vi "UI (The Advanced).vi"() -> ()   [LabVIEW 2017, in "UI.lvlib"]
doc: "The Queued Message Handler of a Worker."
uses:
  UI.lvlib
  _support/Analysis Window Type.ctl
  _support/UI State.ctl
  1af51285-6659-428e-9c15-de70f1a207c9.vi
  1756710f-d813-4077-a3f9-6f06171a4225.vi
  b1498353-a107-4479-98d0-7e76c0451ff6.vi
  242d01f8-d211-4c25-bb6c-8191a2acbe42.vi
  da0d510b-1f54-4e49-9d1f-893e7e8abfcf.vi
  e403ca69-710b-4b23-8527-f02bfa86df9b.vi
  <userlib>/_NEVSTOP/Communicable State Machine(CSM)/AdvanceAPI/CSM - Revert Arguments-Safe String.vi
  <userlib>/_NEVSTOP/Communicable State Machine(CSM)/_Shared/Trim Single-line Text.vi
  <userlib>/_NEVSTOP/Communicable State Machine(CSM)/AdvanceAPI/CSM - Make String Arguments Safe.vi
  <userlib>/_NEVSTOP/Communicable State Machine(CSM)/AdvanceAPI/CSM - Break Down Multiple States String.vi
  <userlib>/_NEVSTOP/Communicable State Machine(CSM)/AdvanceAPI/CSM - Keywords.vi
  <userlib>/_NEVSTOP/Communicable State Machine(CSM)/addons/INI-Static-Variable-Support/_Support/instances/_CSM - Read File Logger Configuration - v1.0.vi
  <userlib>/_NEVSTOP/Communicable State Machine(CSM)/addons/API-String-Arugments-Support/_Support/Convert API String Arguments to Data(variant).vi
  <userlib>/_NEVSTOP/Communicable State Machine(CSM)/addons/API-String-Arugments-Support/_Support/Query Data as API String Arguments(variant).vi
  <userlib>/_NEVSTOP/Communicable State Machine(CSM)/addons/MassData-Parameter/_support/FGV-MassData(lvlibp).vi
  <userlib>/_NEVSTOP/Communicable State Machine(CSM)/_Polymophic/Add State(s) to Queue By BOOL(Element).vi
  <userlib>/_NEVSTOP/Communicable State Machine(CSM)/_Polymophic/CSM - Replace Marks in Messages.vi
  Acquisition/Acquisition.lvlib
  Logging/Logging.lvlib
  <userlib>/_NEVSTOP/Communicable State Machine(CSM)/Communicable State Machine.lvlib
  <userlib>/_NEVSTOP/Communicable State Machine(CSM)/addons/MassData-Parameter/CSM MassData Parameter Support.lvlib
  <userlib>/_NEVSTOP/Communicable State Machine(CSM)/addons/INI-Static-Variable-Support/INI-Static-Variable-Support.lvlib
  Algorithm/Algorithm.lvlib
  <userlib>/_NEVSTOP/Communicable State Machine(CSM)/addons/Logger/CSM File Logger.lvlib
  <userlib>/_NEVSTOP/Communicable State Machine(CSM)/addons/Watchdog/CSM Watchdog.lvlib
  SoundInput-DAQ/SoundInput-DAQ.lvlib
  <userlib>/_NEVSTOP/Communicable State Machine(CSM)/_Polymophic/Build Synchronous Message with Arguments.vi
panel:
  in  "Data Source":enum16{"Simulated Waveform", "Sound Card"}(ring) caption="Data Source: \nSelect Before Running"
  out "WaveformGraph":waveform(dbl)[](graph)
  in  "Analysis Window 1":T1
  out "AnalysisWnd 1":cluster{"f0":dbl, "df":dbl, "magnitude":dbl[]}[](graph)
  in  "Analysis Window 2":T1
  out "AnalysisWnd 2":cluster{"f0":dbl, "df":dbl, "magnitude":dbl[]}[](graph)
  in  "Settings":bool
  in  "Start":bool
  in  "Stop":bool
  out "Status":string
  in  "Exit":bool
  # "Continuous Measurement and Data Logger - CSM Version"
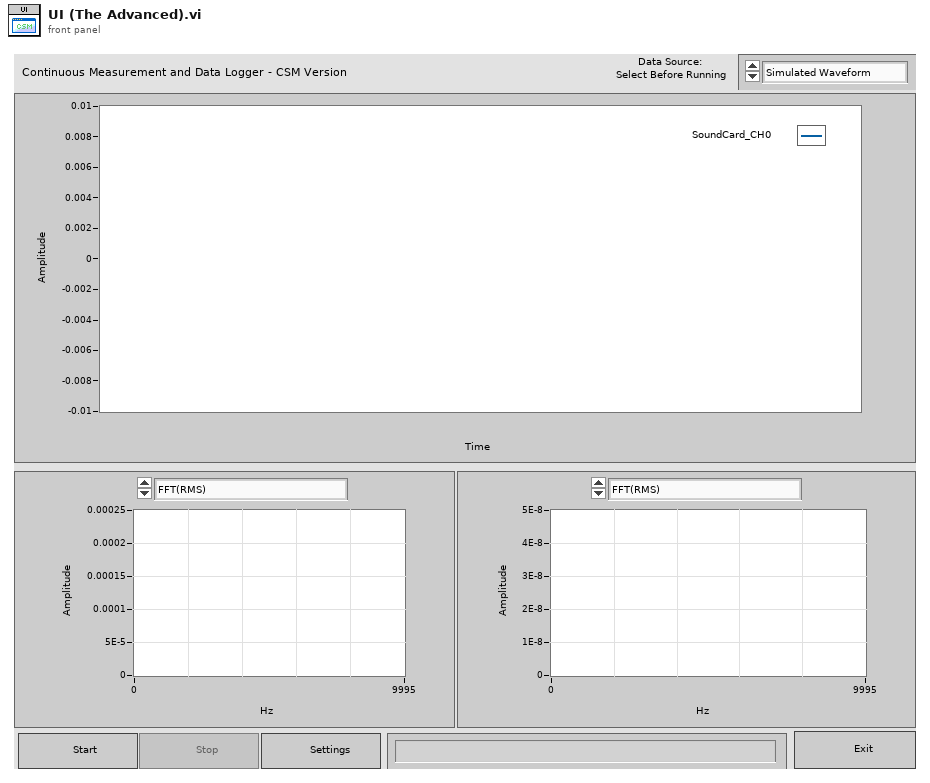
[diagram p1: front panel]
types:
  T1 = typedef "UI.lvlib/Analysis Window Type.ctl" = enum16{"FFT(RMS)", "FFT(Peak)", "Power Spectrum"}
  T2 = cluster{"Enable":bool, "Limit":cluster{"FileSize":i64, "FileNum":i32}, "Timestamp.Format":string, "AutoExit":bool}
  T3 = enum32{"Invalid", "Standard", "Closed", "Hidden", "Minimized", "Maximized"}
  T4 = enum32{"invalid app kind", "Development System", "Run Time System", "Student Edition", "Embedded LabVIEW", "Evaluation", "Custom"}
  T5 = typedef "UI.lvlib/UI State.ctl" = enum16{"Idle", "Acquiring and Logging", "Waiting for Exit", "Waiting for Exit (Acq Stopped)", "Waiting for Exit (Log Stopped)", "Waiting for Stop", "Waiting for Stop (Acq Stopped)", "Waiting for Stop (Log Stopped)"}
  T6 = enum32{"Invalid", "Default", "Floating", "Floating/Auto-Hide", "Modal"}
  T7 = typedef "Communicable State Machine.lvlib/_CSM_Response Source Message.ctl" = cluster{"‘State":string, "’Arguments":string, "’Error":errorcluster}
  T8 = cluster{"Current VI Reference":refnum<vi>, "Close Panel on Exit?":bool}
  T9 = cluster{"Core":cluster{"Current VI Reference":refnum<vi>, "Close Panel on Exit?":bool}, "UI Refs":cluster{"Start Ref":refnum<vi>, "Stop Ref":refnum<vi>, "Settings Ref":refnum<vi>, "Exit Ref":refnum<vi>, "Status Ref":refnum<vi>, "Data Ref":refnum<vi>, "Data Source Ref":refnum<vi>}, "State":T5, "Relationships":string}
  T10 = cluster{"Start Ref":refnum<vi>, "Stop Ref":refnum<vi>, "Settings Ref":refnum<vi>, "Exit Ref":refnum<vi>, "Status Ref":refnum<vi>, "Data Ref":refnum<vi>, "Data Source Ref":refnum<vi>}
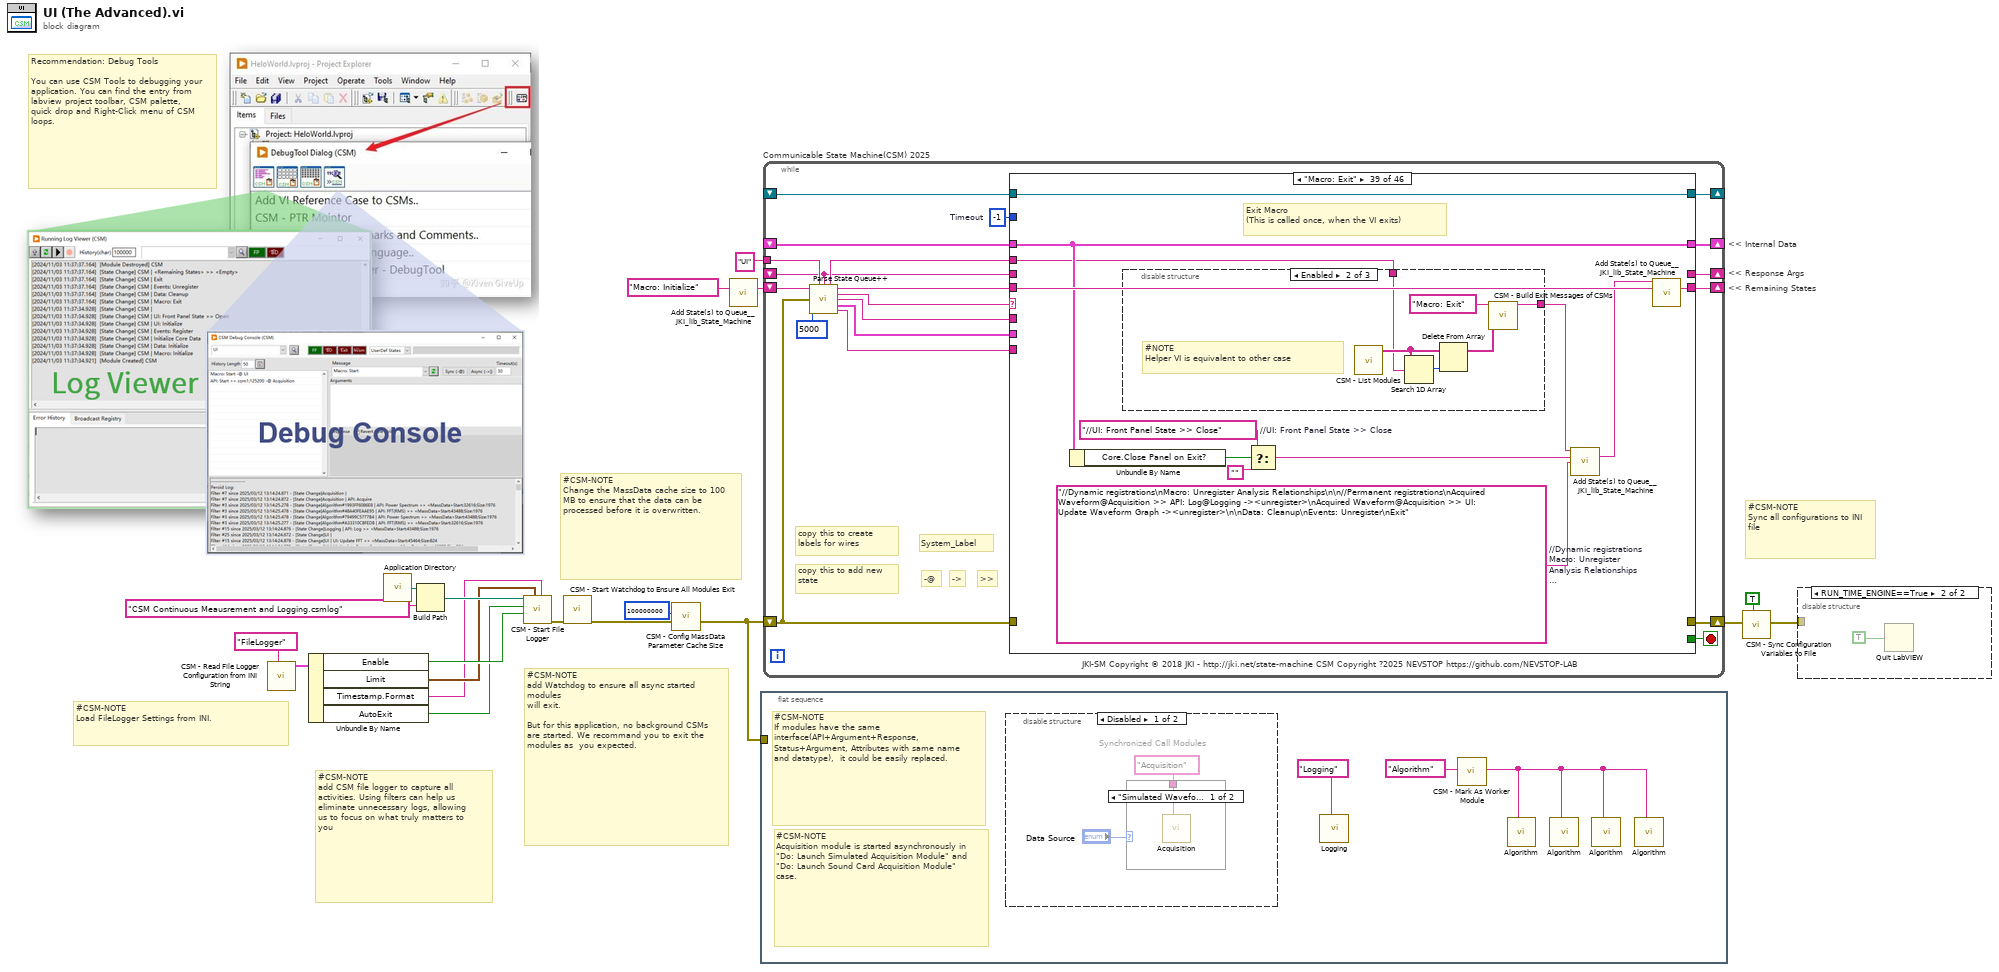
[diagram p0: block diagram]
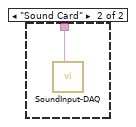
[diagram p3: hidden frame]
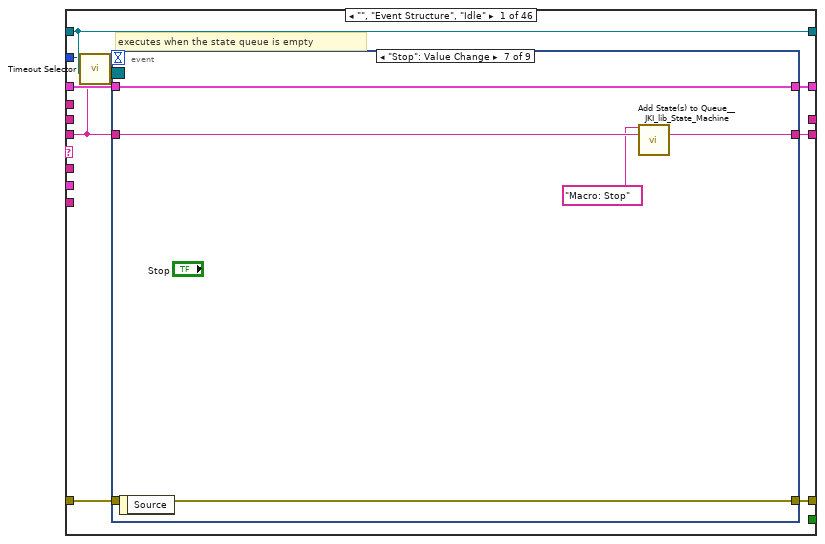
[diagram p5: hidden frame]
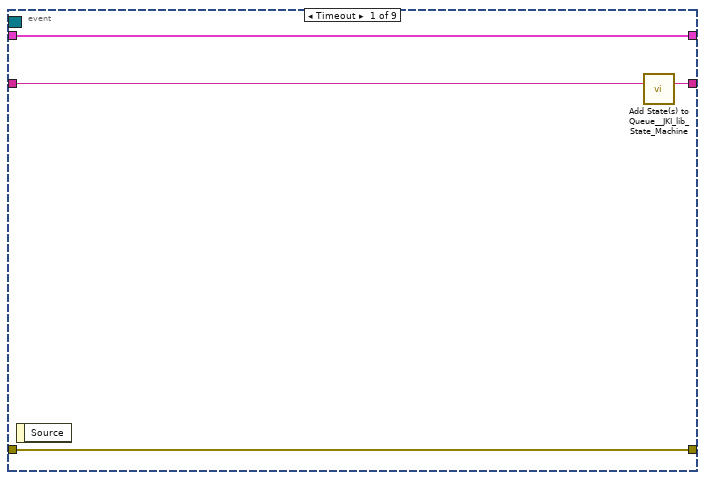
[diagram p6: hidden frame]
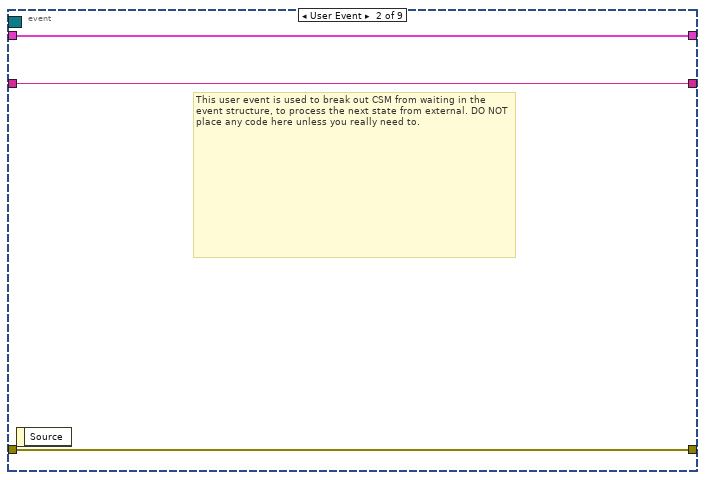
[diagram p7: hidden frame]
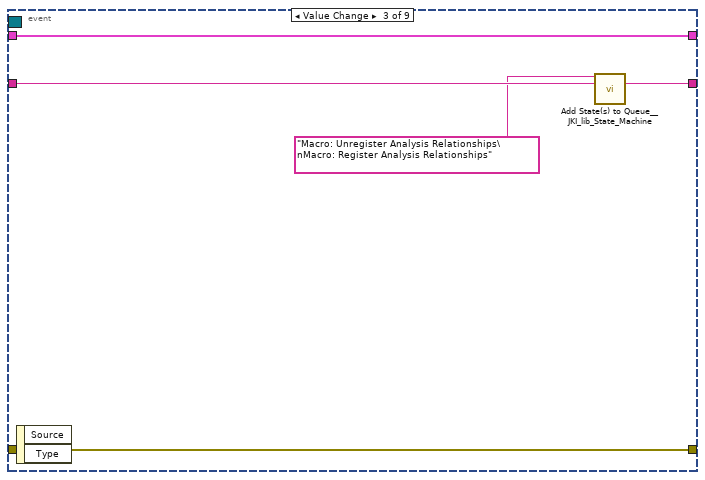
[diagram p8: hidden frame]
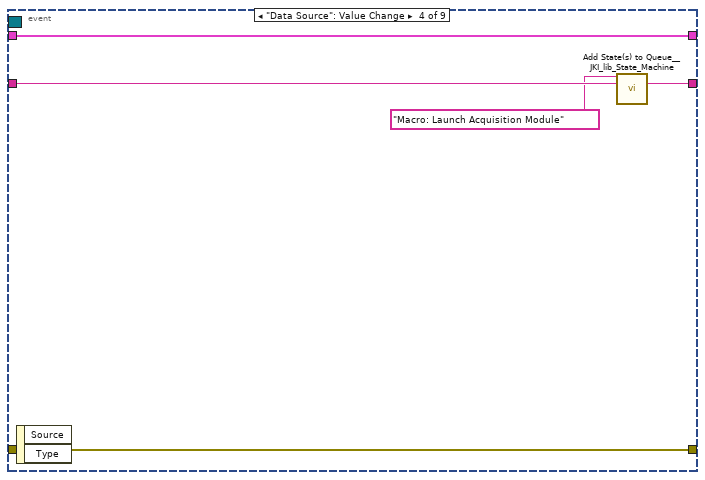
[diagram p9: hidden frame]
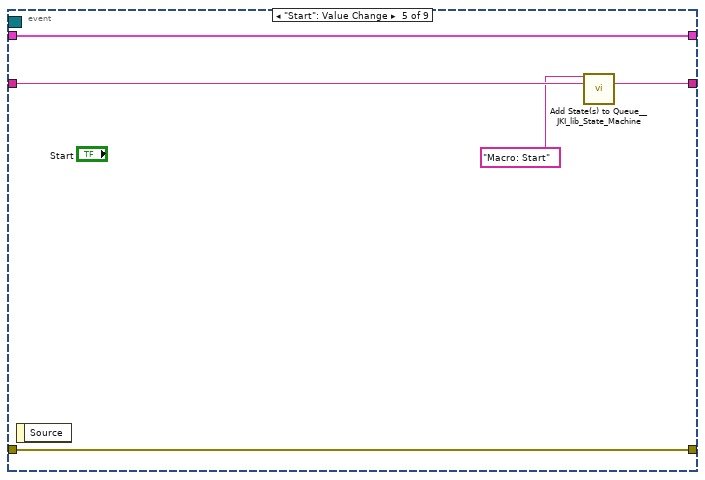
[diagram p10: hidden frame]
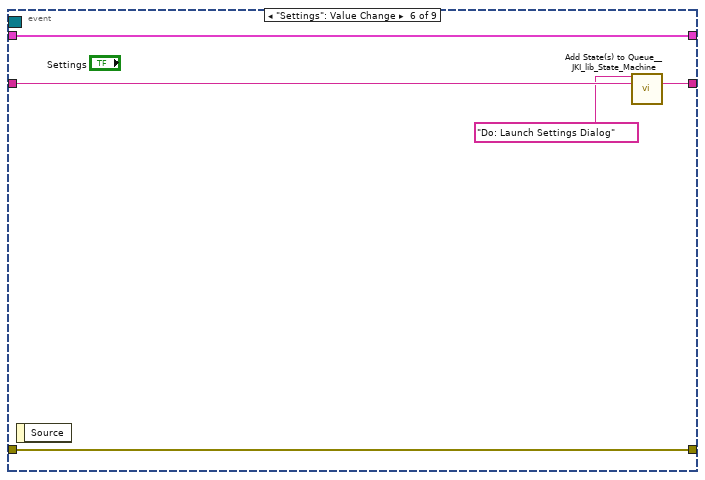
[diagram p11: hidden frame]
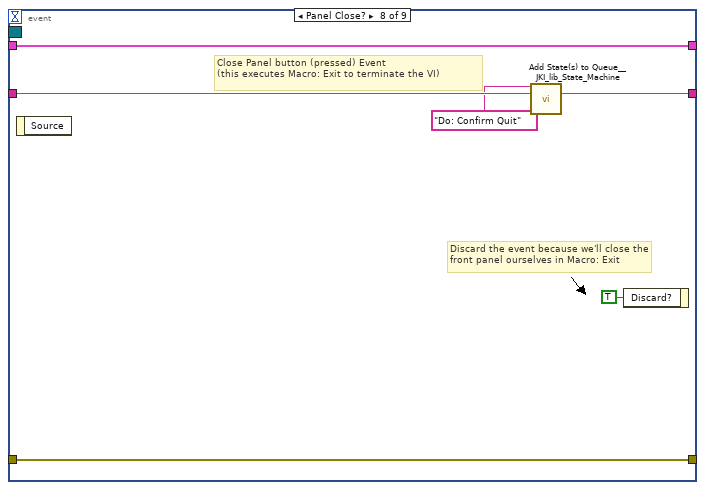
[diagram p12: hidden frame]
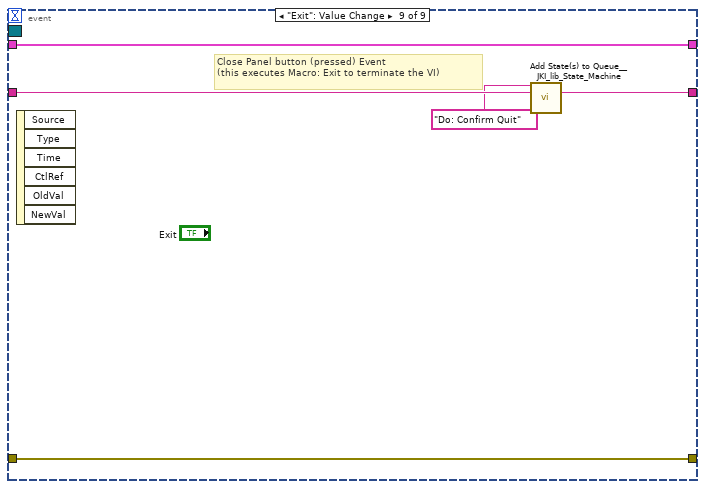
[diagram p13: hidden frame]
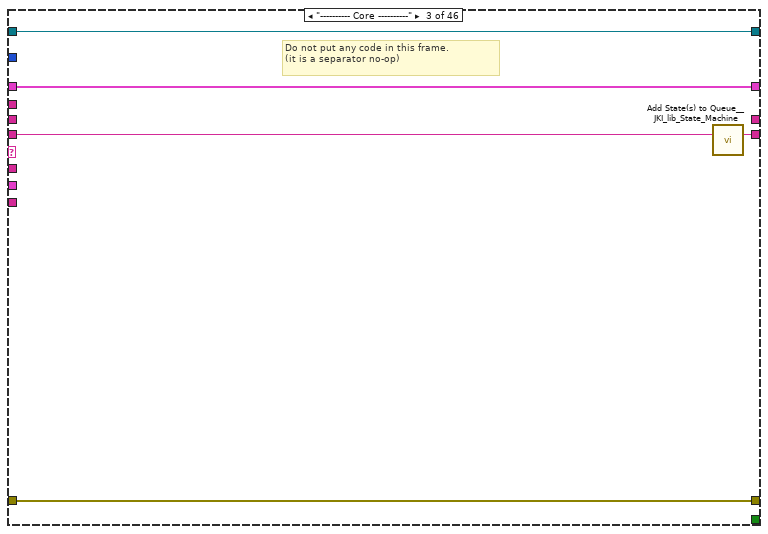
[diagram p15: hidden frame]
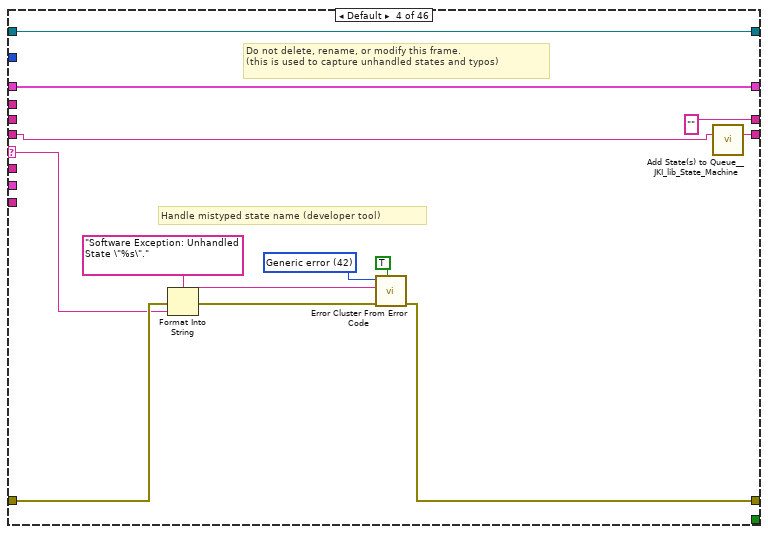
[diagram p16: hidden frame]
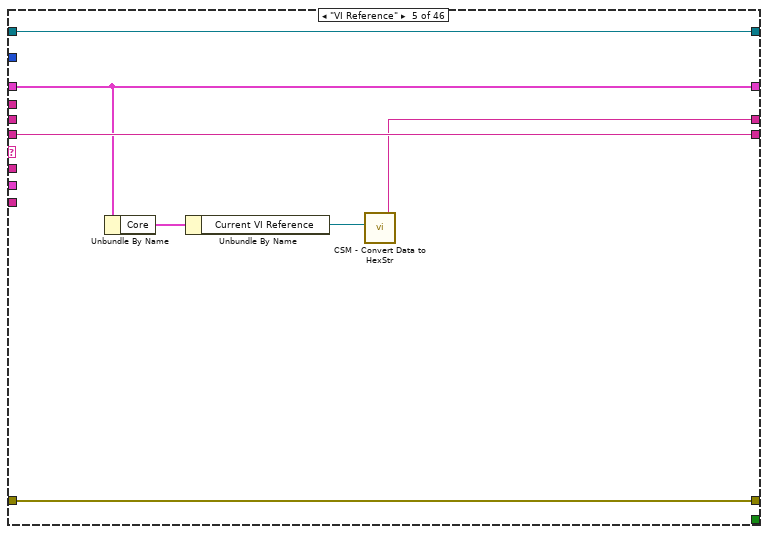
[diagram p17: hidden frame]
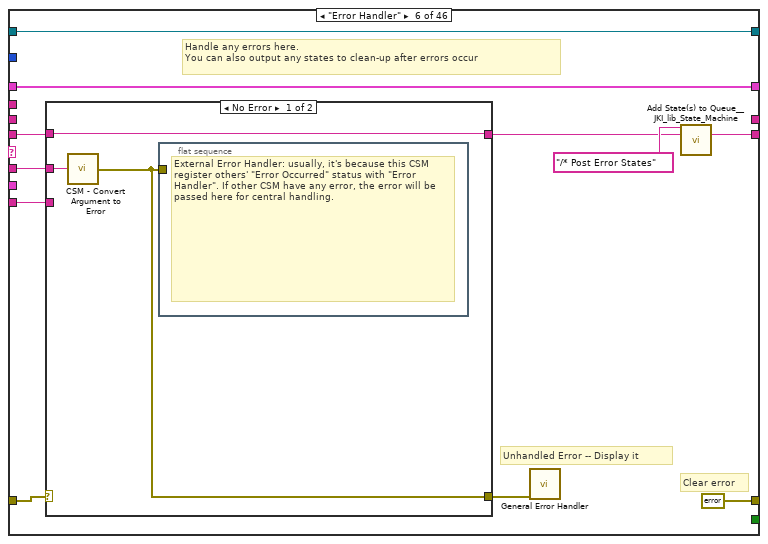
[diagram p18: hidden frame]
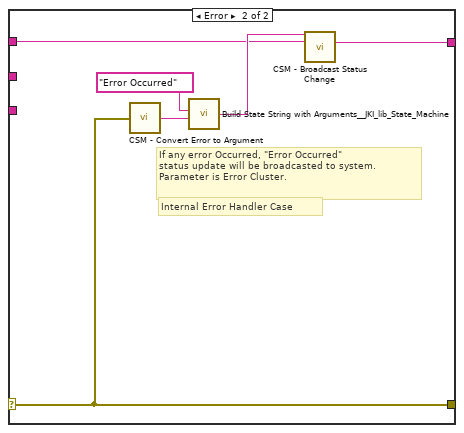
[diagram p19: hidden frame]
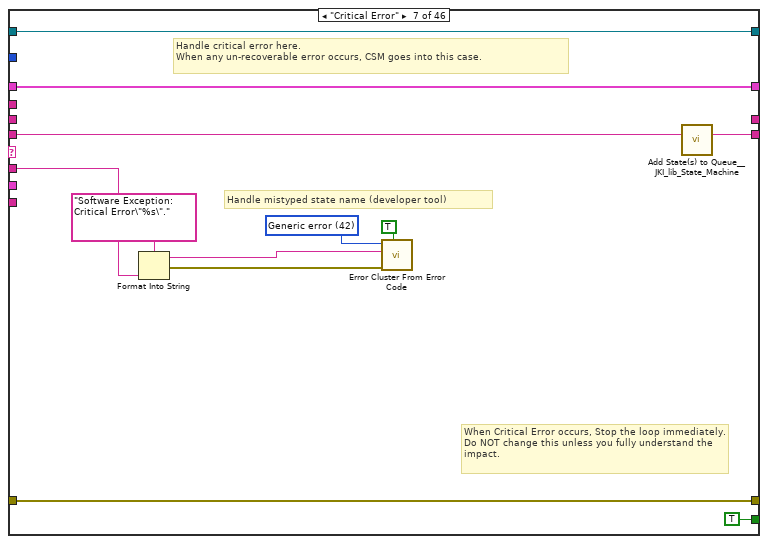
[diagram p20: hidden frame]
diagram:
  # "#CSM-NOTE\nSync all configurations to INI file"
  # "#CSM-NOTE\nChange the MassData cache size to 100 MB to ensure that the data can be processed before it is overwritten."
  # "Recommendation: Debug Tools\n\nYou can use CSM Tools to debugging your application. You can find the entry from labview project toolbar, CSM palette, quick drop and Right-Click menu of CSM loops."
  # "#CSM-NOTE\nLoad FileLogger Settings from INI."
  # "#CSM-NOTE\nadd CSM file logger to capture all activities. Using filters can help us eliminate unnecessary logs, allowing us to focus on what truly matters to you"
  # "#CSM-NOTE\nadd Watchdog to ensure all async started modules\nwill exit. \n\nBut for this application, no background CSMs are started. We recommand you to exit the modules as  you expected."
  # "<< Internal Data"
  # "<< Response Args"
  # "<< Remaining States"
  n1 = call-poly <userlib>:"CSM - Read File Logger Configuration from INI String.vi"("Section Name(\"FileLogger\")"="FileLogger" ("Section Name(\"\" as Default)")) -> ("FileLogger Configuration-v1"=w11:T2)  [unwired: 7 in, 1 out]
  n2 = Unbundle By Name(w11) -> ("Enable"=w10:bool, "Limit"=w9:cluster{"FileSize":i64, "FileNum":i32}, "Timestamp.Format"=w7:string, "AutoExit"=w8:bool)
  n3 = call <vilib>:"Application Directory.vi"() -> ("Application Directory"=w16:path)
  n4 = Build Path(base path=w16, name or relative path="CSM Continuous Meausrement and Logging.csmlog") -> (appended path=w14:path)
  n5 = call <userlib>:"CSM - Start File Logger.vi"("Timestamp Format"=w7, "Log Limit"=w9, "Watchdog? (T)"=w10, "Exit When All Module Exist? (F)"=w8, "Log File Path"=w14) -> ("error out"=w13:errorcluster)  [unwired: 4 in, 2 out]
  n6 = call <userlib>:"CSM - Start Watchdog to Ensure All Modules Exit.vi"("error in (no error)"=w13) -> ("error out"=w5:errorcluster)  [unwired: 10 in]
  n7 = call <userlib>:"CSM - Config MassData Parameter Cache Size.vi"("Error in"=w5, "Size (50M)"=100000000 ("size(1M)")) -> ("Error out"=w4:errorcluster)  [unwired: 9 in]
  n8 = call <vilib>:"Add State(s) to Queue__JKI_lib_State_Machine.vi"("State(s) in (\"\")"="Macro: Initialize") -> ("States Out"=w17:string)  [unwired: 14 in]
  n9 = flat-sequence {
    tunnel: w4 -> [_]
    frame #0 {
      # "#CSM-NOTE\nAcquisition module is started asynchronously in \"Do: Launch Simulated Acquisition Module\" and \"Do: Launch Sound Card Acquisition Module\" case."
      # "#CSM-NOTE\nIf modules have the same interface(API+Argument+Response, Status+Argument, Attributes with same name and datatype),  it could be easily replaced."
      n10 = disable-structure shown="Disabled" {
        frame Disabled {
          # "Synchronized Call Modules"
          n11 = case shown="\"Simulated Waveform\", Default" "Data Source" {
            tunnel: "Acquisition" ("Name(\"\" to use uuid)") -> [w25 w26]
            frame "Simulated Waveform", Default {
              n12 = call "Acquisition.vi"("Name(\"\" to use uuid)"=w25) -> ()  [unwired: 11 in]
            }
            frame "Sound Card" {
              n13 = call "SoundInput-DAQ.vi"("Name(\"\" to use uuid)"=w26) -> ()  [unwired: 11 in]
            }
          }
        }
        frame Enabled {
        }
      }
      n14 = call "Logging.vi"("Name(\"\" to use uuid)"="Logging" ("Name(\"\" to use uuid)")) -> ()  [unwired: 11 in]
      n15 = call <userlib>:"CSM - Mark As Worker Module.vi"("CSM Name"="Algorithm" ("Name(\"\" to use uuid)")) -> ("CSM Name (Marked As Worker)"=w20:string)  [unwired: 9 in]
      n16 = call "Algorithm.vi"("Name(\"\" to use uuid)"=w20) -> ()  [unwired: 11 in]
      n17 = call "Algorithm.vi"("Name(\"\" to use uuid)"=w20) -> ()  [unwired: 11 in]
      n18 = call "Algorithm.vi"("Name(\"\" to use uuid)"=w20) -> ()  [unwired: 11 in]
      n19 = call "Algorithm.vi"("Name(\"\" to use uuid)"=w20) -> ()  [unwired: 11 in]
    }
  }
  n20 = while "Communicable State Machine(CSM) 2025" {
    shift-right: [w41] -> _
    shift-left: _ -> [w40]
    shift-right: [w44] -> w2
    shift-left: w4 -> [w38]
    shift-right: [w43] -> _
    shift-left: w17 -> [w45]
    tunnel: "UI" ("Name(\"\" to use uuid)") -> [w33]
    shift-right: [w36] -> _
    shift-left: _ -> [w28]
    shift-right: [w35] -> _
    shift-left: _ -> [w34]
    stop <- w42 stop-if-true
    w39 = -1  # Timeout
    # "JKI-SM Copyright © 2018 JKI - http://jki.net/state-machine CSM Copyright ?2025 NEVSTOP https://github.com/NEVSTOP-LAB"
    # "copy this to add new state"
    # ">>"
    # "->"
    # "-@"
    # "copy this to create labels for wires"
    # "System_Label"
    n21 = call <userlib>:"Parse State Queue++.vi"("State Queue"=w45, "Name (\"\" to Use UUID)"=w33, "Response Arguments"=w28, "Previous Error"=w38, "Response Timeout (-2 Use Global Settings)"=5000 ("Response Timeout(1000ms)")) -> ("Name Used"=w29:string, "Remaining States"=w46:string, "Current State"=w32:string, "Arguments"=w27:string, "Additional Information"=w31:T7, "Source CSM"=w30:string)  [unwired: 5 in]
    n22 = case shown="\"Macro: Exit\"" w32 {
      selector: w32 -> [_ _ _ w110 _ _ _ _ _ _ _ _ _ _ _ _ _ _ _ _ _ _ _ _ _ _ _ _ _ _ _ _ _ _ _ _ _ _ _ _ _ _ _ _ _ _]
      tunnel: w46 -> [w47 w101 w107 w114 w126 w131 w157 w167 w180 w188 w192 w207 w214 w219 w228 w234 w241 w248 w253 w259 w263 w269 w290 w302 w315 w323 w339 w413 w422 w435 w442 w447 w454 w459 w473 w481 w492 w503 w521 w546 w552 w560 w598 w623 w644 w659]
      tunnel: w27 -> [_ _ _ _ _ w129 w150 w163 w176 _ _ _ _ _ _ w232 w238 _ _ _ _ _ _ _ _ w318 w333 w408 w426 w432 w439 _ _ _ _ _ _ _ _ _ w547 _ _ _ _ _]
      tunnel: w40 -> [w54 w100 w104 w112 w125 w137 w158 w165 w178 w187 w191 w200 w212 w216 _ w231 w239 w243 w250 w258 w262 w266 w276 w292 w305 w321 w335 w411 w428 w434 w441 w444 w451 w462 w476 w488 w495 w499 w519 w543 w549 w553 w593 w622 w643 w658]
      tunnel: [w53 w102 w105 w116 w127 errorcluster {"status"=FALSE, "code"=0, "source"=""} ("error out") w159 errorcluster {"status"=FALSE, "code"=0, "source"=""} ("error out") errorcluster {"status"=FALSE, "code"=0, "source"=""} ("error out") w189 w193 w204 w211 w217 w222 w230 w237 w244 w251 w254 w261 w267 w288 w303 w316 w319 w336 w405 w424 w431 w438 w445 w452 w463 w477 w490 w498 w507 _ w544 w550 w554 _ w615 w631 w646] -> w44
      tunnel: w38 -> [w52 w102 w105 w115 w127 w135 w159 w168 w181 w189 w193 w204 w211 w217 w222 _ _ w245 w251 _ w264 w267 w288 w303 w316 w320 w337 _ _ _ _ w445 w452 w463 w477 w490 w498 w507 _ w544 w550 _ _ _ _ _]
      tunnel: [w55 w101 w106 w113 w126 w133 w156 w166 w179 w188 w192 w206 w213 w218 w227 w234 w241 w247 w252 w259 w263 w268 w289 w302 w315 w322 w338 w413 w423 w435 w442 w446 w453 w460 w474 w482 w493 w504 w520 w545 w551 w560 w591 w623 w644 w659] -> w43
      tunnel: [_ _ _ _ _ _ TRUE _ _ _ _ _ TRUE _ _ _ _ _ _ _ _ _ _ _ _ _ _ _ _ _ _ _ _ _ _ _ _ _ _ _ _ _ _ _ _ _] -> w42
      tunnel: [w51 w100 w104 w112 w125 w137 w158 w165 w178 w187 w191 w205 w212 w216 w221 w229 w235 w243 w250 w258 w262 w266 w275 w292 w305 w321 w335 w411 w428 w434 w441 w444 w451 w462 w472 w479 w494 w505 w519 w543 w549 w553 w592 w622 w643 w658] -> w41
      tunnel: w39 -> [w49 _ _ _ _ _ _ _ _ _ _ _ _ _ _ _ _ _ _ _ _ _ _ _ _ _ _ _ _ _ _ _ _ _ _ _ _ _ _ _ _ _ _ _ _ _]
      tunnel: w30 -> [_ _ _ _ _ w128 _ _ _ _ _ _ _ _ _ _ _ _ _ _ _ _ _ _ _ _ _ _ _ _ _ _ _ _ _ _ _ _ _ _ _ _ _ _ _ _]
      tunnel: w31 -> [_ _ _ _ _ _ _ _ _ _ _ _ _ _ _ _ _ _ _ _ _ _ _ _ _ _ _ _ _ _ _ _ _ _ _ _ _ _ _ _ _ _ _ _ _ _]
      tunnel: [_ _ _ "" w121 _ _ _ _ _ _ _ _ _ _ _ w236 _ _ _ _ _ _ _ _ _ _ _ _ _ _ _ _ _ _ _ _ _ _ _ _ _ _ _ _ _] -> w36
      tunnel: [w50 w99 w103 w108 w124 w136 w148 w162 w175 w186 w190 w194 w209 w215 w225 w233 w240 w242 w249 w257 w260 w265 w287 w301 w314 w317 w332 w412 w427 w433 w440 w443 w450 w461 w475 w489 w497 w506 w512 w542 w548 w561 w597 w621 w642 w657] -> w35
      tunnel: w34 -> [w50 w99 w103 w108 w124 w136 w148 w162 w175 w186 w190 w194 w209 w215 w225 w233 w240 w242 w249 _ w260 w265 w287 w301 w314 w317 w332 w412 w427 w433 w440 w443 w450 w461 w475 w489 w497 w506 w512 w542 w548 w561 w597 w621 w642 w657]
      tunnel: w29 -> [_ _ _ _ _ _ _ _ _ _ _ _ _ _ _ _ _ _ _ w256 _ _ _ _ _ _ _ _ _ _ _ _ _ _ _ _ _ _ w510 _ _ w556 _ w618 _ _]
      tunnel: w28 -> [_ _ _ _ _ _ _ _ _ _ _ _ _ _ _ _ _ _ _ _ _ _ _ _ _ _ _ _ _ _ _ _ _ _ _ _ _ _ _ _ _ _ _ _ _ _]
      frame "", "Event Structure", "Idle" {
        # "executes when the state queue is empty"
        n23 = call <userlib>:"Timeout Selector.vi"("Remaining States"=w47, "Timeout Expected"=w49) -> ("Timeout"=w48:i32)  [unwired: 5 in]
        n24 = event shown="[6] \"Stop\": Value Change" {
          selector: w50 -> [_ _ _ _ _ _ _ _ _]
          dyn-events: _ -> [_ _ _ _ _ _ _ _ _]
          timeout: w48 -> [_ _ _ _ _ _ _ _ _]
          tunnel: w47 -> [w59 w61 w64 w69 w74 w79 w84 w93 w98]
          tunnel: [w58 w61 w65 w70 w75 w80 w85 w92 w97] -> w55
          tunnel: w54 -> [w56 w62 w66 w71 w76 w81 w86 w90 w95]
          tunnel: [w57 w60 w67 w72 w77 w82 w87 w91 w96] -> w53
          tunnel: w52 -> [w57 w60 w67 w72 w77 w82 w87 w91 w96]
          tunnel: [w56 w62 w66 w71 w76 w81 w86 w90 w95] -> w51
          event Timeout {
            n25 = event-data() -> ()  [unwired: 1 in, 1 out]
            n26 = call <vilib>:"Add State(s) to Queue__JKI_lib_State_Machine.vi"("State(s) in (\"\")"=w59) -> ("States Out"=w58:string)  [unwired: 14 in]
          }
          event User Event {
            # "This user event is used to break out CSM from waiting in the event structure, to process the next state from external. DO NOT place any code here unless you really need to."
            n27 = event-data() -> ()  [unwired: 1 in, 1 out]
          }
          event Value Change {
            n28 = event-data() -> ()  [unwired: 1 in, 2 out]
            n29 = call <vilib>:"Add State(s) to Queue__JKI_lib_State_Machine.vi"("State(s) in Front (\"\")"="Macro: Unregister Analysis Relationships\nMacro: Register Analysis Relationships" ("State(s) in Front (\"\")"), "State(s) in (\"\")"=w64) -> ("States Out"=w65:string)  [unwired: 13 in]
          }
          event "Data Source": Value Change {
            n30 = event-data() -> ()  [unwired: 1 in, 2 out]
            n31 = call <vilib>:"Add State(s) to Queue__JKI_lib_State_Machine.vi"("State(s) in Front (\"\")"="Macro: Launch Acquisition Module" ("State(s) in Front (\"\")"), "State(s) in (\"\")"=w69) -> ("States Out"=w70:string)  [unwired: 13 in]
          }
          event "Start": Value Change {
            n32 = event-data() -> ()  [unwired: 1 in, 1 out]
            n33 = call <vilib>:"Add State(s) to Queue__JKI_lib_State_Machine.vi"("State(s) in Front (\"\")"="Macro: Start" ("State(s) in Front (\"\")"), "State(s) in (\"\")"=w74) -> ("States Out"=w75:string)  [unwired: 13 in]
          }
          event "Settings": Value Change {
            n34 = event-data() -> ()  [unwired: 1 in, 1 out]
            n35 = call <vilib>:"Add State(s) to Queue__JKI_lib_State_Machine.vi"("State(s) in Front (\"\")"="Do: Launch Settings Dialog" ("State(s) in Front (\"\")"), "State(s) in (\"\")"=w79) -> ("States Out"=w80:string)  [unwired: 13 in]
          }
          event "Stop": Value Change {
            n36 = event-data() -> ()  [unwired: 1 in, 1 out]
            n37 = call <vilib>:"Add State(s) to Queue__JKI_lib_State_Machine.vi"("State(s) in Front (\"\")"="Macro: Stop" ("State(s) in Front (\"\")"), "State(s) in (\"\")"=w84) -> ("States Out"=w85:string)  [unwired: 13 in]
          }
          event Panel Close? {
            # "Discard the event because we'll close the front panel ourselves in Macro: Exit"
            # "Close Panel button (pressed) Event\n(this executes Macro: Exit to terminate the VI)"
            n38 = event-data() -> ()  [unwired: 1 in, 1 out]
            n39 = call <vilib>:"Add State(s) to Queue__JKI_lib_State_Machine.vi"("State(s) in Front (\"\")"="Do: Confirm Quit", "State(s) in (\"\")"=w93) -> ("States Out"=w92:string)  [unwired: 13 in]
            n40 = event-data("Discard?"=TRUE) -> ()  [unwired: 1 in, 1 out]
          }
          event "Exit": Value Change {
            # "Close Panel button (pressed) Event\n(this executes Macro: Exit to terminate the VI)"
            n41 = event-data() -> ()  [unwired: 1 in, 6 out]
            n42 = call <vilib>:"Add State(s) to Queue__JKI_lib_State_Machine.vi"("State(s) in Front (\"\")"="Do: Confirm Quit", "State(s) in (\"\")"=w98) -> ("States Out"=w97:string)  [unwired: 13 in]
          }
        }
      }
      frame "CSM Documentation" {
        # "CSM Documentation"
        # "State Syntax:\nStateCategory: State >> Argument -@ CSMName\nStateCategory: State >> Argument -> CSMName\n\nLine Terminator: Line feed"
        # "Commenting:\nTo add a comment use \"//\" or \"#\" and all text to the right will be ignored\nCommenting Example:\nUI: Initialize // This initializes the UI\n// Another comment line"
        # "Example:\nUI: Help >> About -@Main\nUI: Help >> About ->Main\n\nWhere \"UI\" is the state category\nWhere \"Help\" is the state\nWhere \"About\" is the argument\nWhere \"Main\" is the Name of CSM,which actually run the \"UI: Help >> About\"\n\n    \"-@\" stands for sync state. Current CSM will wait until the state is finished. \n            - if \"Main\" named CSM does not exist, \"Target Error\" will occur.\n            - if \"Main\" named CSM is in another sync remote state, \"Target Busy Error\" will occur.\n            - if \"Main\" named CSM could not finish the state in time, \"Target Timeout Error\" will occur.\n            - if everything is right. \"Response\" will occur with Argument back from \"Main\" named CSM. \n\n    \"->\" stands for async state. Current CSM will post the state and continue to next state in next iteration.\n            - if \"Main\" named CSM does not exist, \"Target Error\" will occur.\n            - if everything is right. \"Async Message Posted\" will occur.\n            - After State is finished. Caller will receive a \"Async Response\" state from callee.\n\nWhen duplicated name is used for multiple CSM module or some framework problem happens, \"Critical Error\" will occur."
      }
      frame "---------- Core ----------" {
        # "Do not put any code in this frame.\n(it is a separator no-op)"
        n43 = call <vilib>:"Add State(s) to Queue__JKI_lib_State_Machine.vi"("State(s) in (\"\")"=w107) -> ("States Out"=w106:string)  [unwired: 14 in]
      }
      frame Default {
        w119 = 42 items=["No error", "Argument error", "Memory is full", "Out of zone", "End of file", "File already open", "Generic file I/O error", "File not found", "File permission error", "Disk is full", "Duplicate path", "Too many files open", "System feature not enabled", "Resource file not found", "Cannot add resource", "Resource not found", "Image not found", "Image memory error", "Pen does not exist", "Config type invalid", "Config token not found", "Config parse error", "Config memory error", "Bad external code format", "Bad external code offset", "External code not present", "Null window", "Destroy window error", "Null menu", "Print aborted", "Bad print record", "Print driver error", "Windows error during printing", "Memory error during printing", "Print dialog error", "Generic print error", "Invalid device refnum", "Device not found", "Device parameter error", "Device unit error", "Cannot open device", "Device call aborted", "Generic error", "Cancelled by user", "Object ID too low", "Object ID too high", "Object not in heap", "Unknown heap", "Unknown object (invalid DefProc)", "Unknown object (DefProc not in table)", "Message out of range", "Invalid (null) method", "Unknown message", "Manager call not supported", "Bad address", "Network operation in progress", "Network operation timed out", "Connection is busy", "Network attribute not supported", "Network error", "Address in use", "System out of memory", "Connection aborted", "Connection refused", "Not connected", "Already connected", "Connection closed", "Initialization error (interapplication manager)", "Bad occurrence", "Wait on unbound occurrence handler", "Occurrence queue overflow", "Datalog type conflict", "Unused", "Unrecognized type (interapplication manager)", "Memory corrupt", "Failed to make temporary DLL", "Old CIN version", "Drag socket not found", "Failed to load drop-object", "Failed to register OLE object", "Failed to release OLE object", "Format specifier type mismatch", "Unknown format specifier", "Too few format specifiers", "Too many format specifiers", "Scan failed", "Newer CIN version", "Error converting to variant", "Runtime menu error", "Password tampered", "Variant attribute not found", "Incompatible variant data type", "Event data is not available", "Event Store is not present", "Occurrence is not found", "Event Queue is not created", "Event info is not available", "Refnum passed is NULL", "Error retrieving Class GUID", "Error retrieving CoClass GUID", "Error retrieving TypeLib GUID.", "Bad built application magic bytes.", "Specific driver is different from the specific driver associated with the Logical Name.", "There is no session opened to the class driver.", "Max Error", "MAX - Error with config objects", "MAX - Error loading configuration", "MAX - Group not supported"]
        # "Do not delete, rename, or modify this frame.\n(this is used to capture unhandled states and typos)"
        # "Handle mistyped state name (developer tool)"
        n44 = Format Into String(format string="Software Exception: Unhandled State \"%s\"." ("message"), error in=w115, w110) -> (resulting string=w118:string, error out=w117:errorcluster)  [unwired: 1 in]
        n45 = call <vilib>:"Error Cluster From Error Code.vi"("show call chain? (False)"=TRUE, "error in (no error)"=w117, "error message (\"\")"=w118, "error code (0)"=w119) -> ("error out"=w116:errorcluster)  [unwired: 5 in]
        n46 = call <vilib>:"Add State(s) to Queue__JKI_lib_State_Machine.vi"("State(s) in (\"\")"=w114) -> ("States Out"=w113:string)  [unwired: 14 in]
      }
      frame "VI Reference" {
        n47 = Unbundle By Name(w125) -> ("Core"=w123:T8)
        n48 = Unbundle By Name(w123) -> ("Current VI Reference"=w122:refnum<vi>)
        n49 = call <userlib>:"CSM - Convert Data to HexStr.vi"("Variant"=w122) -> ("HEX String (0-9,A-F)"=w121:string)  [unwired: 8 in]
      }
      frame "Error Handler" {
        # "Unhandled Error -- Display it"
        # "Handle any errors here.\nYou can also output any states to clean-up after errors occur"
        # "Clear error"
        n50 = case shown="No Error" w135 {
          selector: w135 -> [_ w142]
          tunnel: [w140 w144] -> w132
          tunnel: w131 -> [w140 w143]
          tunnel: [w139 w142] -> w130
          tunnel: w129 -> [w141 _]
          tunnel: w128 -> [_ _]
          frame No Error {
            n51 = call <userlib>:"CSM - Convert Argument to Error.vi"("Argument"=w141) -> ("Error"=w139:errorcluster)  [unwired: 4 in]
            n52 = flat-sequence {
              tunnel: w139 -> [_]
              frame #0 {
                # "External Error Handler: usually, it's because this CSM register others' \"Error Occurred\" status with \"Error Handler\". If other CSM have any error, the error will be passed here for central handling."
              }
            }
          }
          frame Error {
            # "Internal Error Handler Case"
            # "If any error Occurred, \"Error Occurred\" \nstatus update will be broadcasted to system.\nParameter is Error Cluster."
            n53 = call <userlib>:"CSM - Convert Error to Argument.vi"("Error"=w142) -> ("Argument"=w146:string)  [unwired: 4 in]
            n54 = call <vilib>:"Build State String with Arguments__JKI_lib_State_Machine.vi"("Arguments (\"\")"=w146, "State"="Error Occurred" ("Status with Arguments")) -> ("State with Arguments"=w145:string)  [unwired: 4 in]
            n55 = call <userlib>:"CSM - Broadcast Status Change.vi"("Status With Arguments"=w145, "State Queue"=w143) -> ("Remaining States"=w144:string)  [unwired: 13 in]
          }
        }
        n56 = call <vilib>:"General Error Handler.vi"("error in (no error)"=w130) -> ()  [unwired: 10 in, 5 out]
        n57 = call <vilib>:"Add State(s) to Queue__JKI_lib_State_Machine.vi"("State(s) in Front (\"\")"="/* Post Error States", "State(s) in (\"\")"=w132) -> ("States Out"=w133:string)  [unwired: 13 in]
      }
      frame "Critical Error" {
        w154 = 42 items=["No error", "Argument error", "Memory is full", "Out of zone", "End of file", "File already open", "Generic file I/O error", "File not found", "File permission error", "Disk is full", "Duplicate path", "Too many files open", "System feature not enabled", "Resource file not found", "Cannot add resource", "Resource not found", "Image not found", "Image memory error", "Pen does not exist", "Config type invalid", "Config token not found", "Config parse error", "Config memory error", "Bad external code format", "Bad external code offset", "External code not present", "Null window", "Destroy window error", "Null menu", "Print aborted", "Bad print record", "Print driver error", "Windows error during printing", "Memory error during printing", "Print dialog error", "Generic print error", "Invalid device refnum", "Device not found", "Device parameter error", "Device unit error", "Cannot open device", "Device call aborted", "Generic error", "Cancelled by user", "Object ID too low", "Object ID too high", "Object not in heap", "Unknown heap", "Unknown object (invalid DefProc)", "Unknown object (DefProc not in table)", "Message out of range", "Invalid (null) method", "Unknown message", "Manager call not supported", "Bad address", "Network operation in progress", "Network operation timed out", "Connection is busy", "Network attribute not supported", "Network error", "Address in use", "System out of memory", "Connection aborted", "Connection refused", "Not connected", "Already connected", "Connection closed", "Initialization error (interapplication manager)", "Bad occurrence", "Wait on unbound occurrence handler", "Occurrence queue overflow", "Datalog type conflict", "Unused", "Unrecognized type (interapplication manager)", "Memory corrupt", "Failed to make temporary DLL", "Old CIN version", "Drag socket not found", "Failed to load drop-object", "Failed to register OLE object", "Failed to release OLE object", "Format specifier type mismatch", "Unknown format specifier", "Too few format specifiers", "Too many format specifiers", "Scan failed", "Newer CIN version", "Error converting to variant", "Runtime menu error", "Password tampered", "Variant attribute not found", "Incompatible variant data type", "Event data is not available", "Event Store is not present", "Occurrence is not found", "Event Queue is not created", "Event info is not available", "Refnum passed is NULL", "Error retrieving Class GUID", "Error retrieving CoClass GUID", "Error retrieving TypeLib GUID.", "Bad built application magic bytes.", "Specific driver is different from the specific driver associated with the Logical Name.", "There is no session opened to the class driver.", "Max Error", "MAX - Error with config objects", "MAX - Error loading configuration", "MAX - Group not supported"]
        # "Handle critical error here.\nWhen any un-recoverable error occurs, CSM goes into this case."
        # "When Critical Error occurs, Stop the loop immediately. Do NOT change this unless you fully understand the impact."
        # "Handle mistyped state name (developer tool)"
        n58 = Format Into String(format string="Software Exception: Critical Error\"%s\"." ("message"), w150) -> (resulting string=w153:string, error out=w152:errorcluster)  [unwired: 2 in]
        n59 = call <vilib>:"Error Cluster From Error Code.vi"("show call chain? (False)"=TRUE, "error in (no error)"=w152, "error message (\"\")"=w153, "error code (0)"=w154) -> ()  [unwired: 5 in, 1 out]
        n60 = call <vilib>:"Add State(s) to Queue__JKI_lib_State_Machine.vi"("State(s) in (\"\")"=w157) -> ("States Out"=w156:string)  [unwired: 14 in]
      }
      frame "Target Timeout Error" {
        w171 = 42 items=["No error", "Argument error", "Memory is full", "Out of zone", "End of file", "File already open", "Generic file I/O error", "File not found", "File permission error", "Disk is full", "Duplicate path", "Too many files open", "System feature not enabled", "Resource file not found", "Cannot add resource", "Resource not found", "Image not found", "Image memory error", "Pen does not exist", "Config type invalid", "Config token not found", "Config parse error", "Config memory error", "Bad external code format", "Bad external code offset", "External code not present", "Null window", "Destroy window error", "Null menu", "Print aborted", "Bad print record", "Print driver error", "Windows error during printing", "Memory error during printing", "Print dialog error", "Generic print error", "Invalid device refnum", "Device not found", "Device parameter error", "Device unit error", "Cannot open device", "Device call aborted", "Generic error", "Cancelled by user", "Object ID too low", "Object ID too high", "Object not in heap", "Unknown heap", "Unknown object (invalid DefProc)", "Unknown object (DefProc not in table)", "Message out of range", "Invalid (null) method", "Unknown message", "Manager call not supported", "Bad address", "Network operation in progress", "Network operation timed out", "Connection is busy", "Network attribute not supported", "Network error", "Address in use", "System out of memory", "Connection aborted", "Connection refused", "Not connected", "Already connected", "Connection closed", "Initialization error (interapplication manager)", "Bad occurrence", "Wait on unbound occurrence handler", "Occurrence queue overflow", "Datalog type conflict", "Unused", "Unrecognized type (interapplication manager)", "Memory corrupt", "Failed to make temporary DLL", "Old CIN version", "Drag socket not found", "Failed to load drop-object", "Failed to register OLE object", "Failed to release OLE object", "Format specifier type mismatch", "Unknown format specifier", "Too few format specifiers", "Too many format specifiers", "Scan failed", "Newer CIN version", "Error converting to variant", "Runtime menu error", "Password tampered", "Variant attribute not found", "Incompatible variant data type", "Event data is not available", "Event Store is not present", "Occurrence is not found", "Event Queue is not created", "Event info is not available", "Refnum passed is NULL", "Error retrieving Class GUID", "Error retrieving CoClass GUID", "Error retrieving TypeLib GUID.", "Bad built application magic bytes.", "Specific driver is different from the specific driver associated with the Logical Name.", "There is no session opened to the class driver.", "Max Error", "MAX - Error with config objects", "MAX - Error loading configuration", "MAX - Group not supported"]
        # "Handle target timeout error here.\nWhen this CSM could not get the sync-call response in time, this CSM goes into this case."
        # "Handle mistyped state name (developer tool)"
        n61 = Format Into String(format string="Software Exception: Target could not finish the \"%s\" state in time." ("message"), error in=w168, w163) -> (resulting string=w170:string, error out=w169:errorcluster)  [unwired: 1 in]
        n62 = call <vilib>:"Error Cluster From Error Code.vi"("show call chain? (False)"=TRUE, "error in (no error)"=w169, "error message (\"\")"=w170, "error code (0)"=w171) -> ("error out"=w160:errorcluster)  [unwired: 5 in]
        n63 = call <vilib>:"General Error Handler.vi"("error in (no error)"=w160) -> ()  [unwired: 10 in, 5 out]
        n64 = call <vilib>:"Add State(s) to Queue__JKI_lib_State_Machine.vi"("State(s) in (\"\")"=w167) -> ("States Out"=w166:string)  [unwired: 14 in]
      }
      frame "Target Error" {
        w184 = 42 items=["No error", "Argument error", "Memory is full", "Out of zone", "End of file", "File already open", "Generic file I/O error", "File not found", "File permission error", "Disk is full", "Duplicate path", "Too many files open", "System feature not enabled", "Resource file not found", "Cannot add resource", "Resource not found", "Image not found", "Image memory error", "Pen does not exist", "Config type invalid", "Config token not found", "Config parse error", "Config memory error", "Bad external code format", "Bad external code offset", "External code not present", "Null window", "Destroy window error", "Null menu", "Print aborted", "Bad print record", "Print driver error", "Windows error during printing", "Memory error during printing", "Print dialog error", "Generic print error", "Invalid device refnum", "Device not found", "Device parameter error", "Device unit error", "Cannot open device", "Device call aborted", "Generic error", "Cancelled by user", "Object ID too low", "Object ID too high", "Object not in heap", "Unknown heap", "Unknown object (invalid DefProc)", "Unknown object (DefProc not in table)", "Message out of range", "Invalid (null) method", "Unknown message", "Manager call not supported", "Bad address", "Network operation in progress", "Network operation timed out", "Connection is busy", "Network attribute not supported", "Network error", "Address in use", "System out of memory", "Connection aborted", "Connection refused", "Not connected", "Already connected", "Connection closed", "Initialization error (interapplication manager)", "Bad occurrence", "Wait on unbound occurrence handler", "Occurrence queue overflow", "Datalog type conflict", "Unused", "Unrecognized type (interapplication manager)", "Memory corrupt", "Failed to make temporary DLL", "Old CIN version", "Drag socket not found", "Failed to load drop-object", "Failed to register OLE object", "Failed to release OLE object", "Format specifier type mismatch", "Unknown format specifier", "Too few format specifiers", "Too many format specifiers", "Scan failed", "Newer CIN version", "Error converting to variant", "Runtime menu error", "Password tampered", "Variant attribute not found", "Incompatible variant data type", "Event data is not available", "Event Store is not present", "Occurrence is not found", "Event Queue is not created", "Event info is not available", "Refnum passed is NULL", "Error retrieving Class GUID", "Error retrieving CoClass GUID", "Error retrieving TypeLib GUID.", "Bad built application magic bytes.", "Specific driver is different from the specific driver associated with the Logical Name.", "There is no session opened to the class driver.", "Max Error", "MAX - Error with config objects", "MAX - Error loading configuration", "MAX - Group not supported"]
        # "Handle target error here.\nWhen this CSM try to communicate with an un-existed CSM, this CSM goes into this case."
        # "Handle mistyped state name (developer tool)"
        n65 = Format Into String(format string="Software Exception: Target \"%s\" does not exists." ("message"), error in=w181, w176) -> (resulting string=w183:string, error out=w182:errorcluster)  [unwired: 1 in]
        n66 = call <vilib>:"Error Cluster From Error Code.vi"("show call chain? (False)"=TRUE, "error in (no error)"=w182, "error message (\"\")"=w183, "error code (0)"=w184) -> ("error out"=w174:errorcluster)  [unwired: 5 in]
        n67 = call <vilib>:"General Error Handler.vi"("error in (no error)"=w174) -> ()  [unwired: 10 in, 5 out]
        n68 = call <vilib>:"Add State(s) to Queue__JKI_lib_State_Machine.vi"("State(s) in (\"\")"=w180) -> ("States Out"=w179:string)  [unwired: 14 in]
      }
      frame "Async Response", "Response" {
        # "Handle Async-call Response (\"Async Response\" for ->)"
        # "Handle Sync-call Response (\"Response\" for -@)"
        # "After Message is executed, CSM+ goes to this state for receive the response. \n    For Async Message(->), \"Async Response\" is used. This CSM will goes to \"Async Message Posted\" immediately and receive the \"Async Response\" after the callee finishes the message.\n    For Sync Message(@),  This CSM will wait until the message is done and immediately goes to \"Response\""
      }
      frame "Async Message Posted" {
        # "Handle post action for async message (->)."
        # "After Async Message is posted (->), CSM+ goes to this state for post-action. You can use Argument - State to tell which Async Message is called."
      }
      frame "Initialize Core Data" {
        # "Do not delete, rename, or modify this frame.\n(this is used to determine panel behavior on exit)"
        # "originally closed?"
        # "exe?"
        # "If panel starts closed or is an EXE, then close it when we exit"
        n69 = property class="VI"() -> ("FP.State"=w197:T3)  [unwired: 2 in, 2 out]
        n70 = property class="App"() -> ("App.Kind"=w203:T4)  [unwired: 2 in, 2 out]
        n71 = control-ref of="Current VI Reference"() -> (w198:refnum<vi>)
        n72 = Equal?(x=w197, y=T3."Closed" ("Front Panel Window:State")) -> (x = y?=w195:bool)
        n73 = Equal?(x=w203, y=T4."Run Time System" ("Application:Kind")) -> (x = y?=w201:bool)
        n74 = Or(x=w195, y=w201) -> (x .or. y?=w199:bool)
        n75 = Bundle By Name(cluster=w200, "Core.Current VI Reference"=w198, "Core.Close Panel on Exit?"=w199) -> (w205:T9)
        n76 = call <vilib>:"Add State(s) to Queue__JKI_lib_State_Machine.vi"("State(s) in (\"\")"=w207) -> ("States Out"=w206:string)  [unwired: 14 in]
      }
      frame "Exit" {
        # "Do not put any code in this frame.\n(No errors that occur here will be handled.)"
        n77 = local write "Status"("Exit" ("Exit String")) -> ()
        n78 = call <vilib>:"Add State(s) to Queue__JKI_lib_State_Machine.vi"("State(s) in (\"\")"=w214) -> ("States Out"=w213:string)  [unwired: 14 in]
      }
      frame "---------- Data ----------" {
        # "Do not put any code in this frame.\n(It is a separator no-op. You can make a copy of this frame to create a new Data frame)"
        n79 = call <vilib>:"Add State(s) to Queue__JKI_lib_State_Machine.vi"("State(s) in (\"\")"=w219) -> ("States Out"=w218:string)  [unwired: 14 in]
      }
      frame "Data: Initialize" {
        w220 = ""  # Relationships
        w223 = UI_State."Idle"  # State
        w224 = T10 {"Start Ref"=refnum, "Stop Ref"=refnum, "Settings Ref"=refnum, "Exit Ref"=refnum, "Status Ref"=refnum, "Data Ref"=refnum, "Data Source Ref"=refnum}  # UI Refs
        w226 = T8 {"Current VI Reference"=refnum, "Close Panel on Exit?"=FALSE}  # Core
        # "Initialize the shift-register data, here.\n(data names are defined by what you wire into the bundle function)"
        n80 = Bundle("Core"=w226, "UI Refs"=w224, "State"=w223, "Relationships"=w220) -> (w221:T9)  [unwired: 1 in]
        n81 = call <vilib>:"Add State(s) to Queue__JKI_lib_State_Machine.vi"("State(s) in (\"\")"=w228) -> ("States Out"=w227:string)  [unwired: 14 in]
      }
      frame "Data: Set Configuration" {
        n82 = call "Convert API String Arguments to Data.vim"("Reference Type"=w231, "API String"=w232) -> ("error out"=w230:errorcluster, "Data"=w229:T9)  [unwired: 6 in]
      }
      frame "Data: Get Configuration", "Data: Get Internal Data" {
        n83 = call "Query Data as API String Arguments.vim"("Name"=w238, "Cluster Data"=w239) -> ("error"=w237:errorcluster, "API String"=w236:string, "Cluster Data (dup)"=w235:T9)  [unwired: 7 in]
      }
      frame "Data: Cleanup" {
        # "Cleanup any data and references, here.\n(this is called automatically, by the Macro: Exit)"
        n84 = Unbundle By Name(w243) -> ("Core.Current VI Reference"=w246:refnum<vi>)
        n85 = Close Reference(reference=w246, error in (no error)=w245) -> (error out=w244:errorcluster)
        n86 = call <vilib>:"Add State(s) to Queue__JKI_lib_State_Machine.vi"("State(s) in (\"\")"=w248) -> ("States Out"=w247:string)  [unwired: 14 in]
      }
      frame "---------- Events ----------" {
        # "Do not put any code in this frame.\n(It is a separator no-op. You can make a copy of this frame to create a new UI frame)"
        n87 = call <vilib>:"Add State(s) to Queue__JKI_lib_State_Machine.vi"("State(s) in (\"\")"=w253) -> ("States Out"=w252:string)  [unwired: 14 in]
      }
      frame "Events: Register" {
        # "Register message event to break Waiting in Event structure."
        n88 = call <userlib>:"CSM - Get New State Notifier Event.vi"("Name (\"\" to Use UUID)"=w256) -> ("error out"=w254:errorcluster, "New State Notifier Event"=w255:refnum<user-event>)  [unwired: 9 in]
        n89 = register-events(w255) -> (reference out=w257:refnum<event-registration>)  [unwired: 2 in, 1 out]
      }
      frame "Events: Unregister" {
        n90 = Unregister For Events(event registration refnum=w260, error in=w264) -> (error out=w261:errorcluster)
      }
      frame "---------- UI ----------" {
        # "Do not put any code in this frame.\n(It is a separator no-op. You can make a copy of this frame to create a new UI frame)"
        n91 = call <vilib>:"Add State(s) to Queue__JKI_lib_State_Machine.vi"("State(s) in (\"\")"=w269) -> ("States Out"=w268:string)  [unwired: 14 in]
      }
      frame "UI: Initialize" {
        w273 = cluster{"f0":dbl, "df":dbl, "magnitude":dbl[]}[] [] ("FFT")
        # "Initialize the User Interface, here.\n(this is called automatically, by the Macro: Init)"
        n92 = control-ref of="WaveformGraph"() -> (w279:refnum<vi>)
        n93 = control-ref of="Start"() -> (w284:refnum<vi>)
        n94 = control-ref of="Stop"() -> (w283:refnum<vi>)
        n95 = control-ref of="Settings"() -> (w285:refnum<vi>)
        n96 = control-ref of="Exit"() -> (w286:refnum<vi>)
        n97 = control-ref of="Status"() -> (w280:refnum<vi>)
        n98 = control-ref of="Data Source"() -> (w270:refnum<vi>)
        n99 = local write "AnalysisWnd 2"(w273) -> ()
        n100 = property on="AnalysisWnd 1" class="WFGraph (strict)"("Value"=w273) -> ()  [unwired: 2 in, 2 out]
        n101 = Bundle By Name(cluster=w276, "UI Refs.Start Ref"=w284, "UI Refs.Stop Ref"=w283, "UI Refs.Settings Ref"=w285, "UI Refs.Exit Ref"=w286, "UI Refs.Status Ref"=w280, "UI Refs.Data Ref"=w279, "UI Refs.Data Source Ref"=w270) -> (w275:T9)
        n102 = Build Array(w284, w286, w285, w270) -> (w282:refnum<vi>[])
        n103 = Build Array(w283) -> (w281:refnum<vi>[])
        n104 = property on="WaveformGraph" class="WFChart (strict)"("History Data"=waveform(dbl)[][] []) -> ()  [unwired: 2 in, 2 out]
        n105 = call "Set Enable State on Multiple Controls.vi"("Enable?"=TRUE, "Controls"=w282) -> ()  [unwired: 10 in]
        n106 = call "Set Enable State on Multiple Controls.vi"("Enable?"=FALSE, "Controls"=w281) -> ()  [unwired: 10 in]
        n107 = local write "Analysis Window 1"(Analysis_Window_Type."FFT(RMS)" ("Analysis Window 1")) -> ()
        n108 = local write "Analysis Window 2"(Analysis_Window_Type."Power Spectrum" ("Analysis Window 2")) -> ()
        n109 = call <vilib>:"Add State(s) to Queue__JKI_lib_State_Machine.vi"("State(s) in (\"\")"=w290) -> ("States Out"=w289:string)  [unwired: 14 in]
      }
      frame "UI: Update When Start" {
        # "Enable: Stop\nDisable: Start, Exit, Settings"
        n110 = Unbundle By Name(w292) -> ("UI Refs.Stop Ref"=w298:refnum<vi>, "UI Refs.Start Ref"=w297:refnum<vi>, "UI Refs.Exit Ref"=w296:refnum<vi>, "UI Refs.Settings Ref"=w295:refnum<vi>, "UI Refs.Data Source Ref"=w291:refnum<vi>)
        n111 = Build Array(w297, w296, w295, w291) -> (w300:refnum<vi>[])
        n112 = Build Array(w298) -> (w299:refnum<vi>[])
        n113 = call "Set Enable State on Multiple Controls.vi"("Enable?"=TRUE, "Controls"=w299) -> ()  [unwired: 10 in]
        n114 = call "Set Enable State on Multiple Controls.vi"("Enable?"=FALSE, "Controls"=w300) -> ()  [unwired: 10 in]
      }
      frame "UI: Update When Stop" {
        # "Enable: Start, Exit, Settings\nDisable: Stop"
        n115 = Unbundle By Name(w305) -> ("UI Refs.Stop Ref"=w310:refnum<vi>, "UI Refs.Start Ref"=w311:refnum<vi>, "UI Refs.Exit Ref"=w312:refnum<vi>, "UI Refs.Settings Ref"=w313:refnum<vi>, "UI Refs.Data Source Ref"=w304:refnum<vi>)
        n116 = Build Array(w311, w312, w313, w304) -> (w308:refnum<vi>[])
        n117 = Build Array(w310) -> (w309:refnum<vi>[])
        n118 = call "Set Enable State on Multiple Controls.vi"("Enable?"=FALSE, "Controls"=w309) -> ()  [unwired: 10 in]
        n119 = call "Set Enable State on Multiple Controls.vi"("Enable?"=TRUE, "Controls"=w308) -> ()  [unwired: 10 in]
      }
      frame "UI: Cursor Set" {
        # "Argument"
        # "Set and Unset Cursor Busy.\n(Usage: \"UI: Cursor Set >> Busy|Idle\")"
        n120 = disable-structure shown="Default" {
          disable-tunnel: w320 -> [w326 w331]
          disable-tunnel: [w325 w331] -> w319
          disable-tunnel: w318 -> [w324 _]
          frame condition #0 (active) {
            n121 = case shown="\"Busy\"" w324 {
              tunnel: w326 -> [w328 w330]
              tunnel: [w327 w329] -> w325
              frame "Idle", Default {
                n122 = call <vilib>:"Unset Busy.vi"("error in (no error)"=w328) -> ("error out"=w327:errorcluster)  [unwired: 10 in]
              }
              frame "Busy" {
                n123 = call <vilib>:"Set Busy.vi"("error in (no error)"=w330) -> ("error out"=w329:errorcluster)  [unwired: 9 in, 1 out]
              }
            }
          }
          frame condition #1 {
          }
        }
        n124 = call <vilib>:"Add State(s) to Queue__JKI_lib_State_Machine.vi"("State(s) in (\"\")"=w323) -> ("States Out"=w322:string)  [unwired: 14 in]
      }
      frame "UI: Front Panel State" {
        # "Argument"
        # "Set Front Panel Open or Closed\n(Usage: \"UI: Front Panel State >> Open|Close\")"
        n125 = Unbundle By Name(w335) -> ("Core.Current VI Reference"=w334:refnum<vi>)
        n126 = case shown="\"Minimize\", \"Minimized\"" w333 {
          tunnel: w337 -> [w345 w360 w371 w384 w397]
          tunnel: [w347 w361 w373 w386 w399] -> w336
          tunnel: w334 -> [w346 w358 w372 w385 w398]
          frame "Open", "Standard", Default {
            w340 = T3."Standard" ("State")
            n127 = property class="VI"(reference=w346, error in=w345) -> (reference out=w343:refnum<vi>, error out=w344:errorcluster, "FP.State"=w342:T3)
            n128 = Not Equal?(x=w342, y=w340) -> (x != y?=w341:bool)
            n129 = case shown="True" w341 {
              tunnel: [w351 w353] -> w347
              tunnel: w344 -> [w350 w353]
              tunnel: w343 -> [w349 _]
              tunnel: w340 -> [w348 _]
              frame True {
                n130 = invoke class="VI" method="FP.Open"(reference=w349, error in=w350, "Activate"=TRUE, "State"=w348) -> (error out=w351:errorcluster)  [unwired: 1 in, 4 out]
              }
              frame False {
              }
            }
          }
          frame "Close", "Closed" {
            n131 = property class="VI"(reference=w358, error in=w360) -> (reference out=w357:refnum<vi>, error out=w359:errorcluster, "FP.State"=w355:T3)
            n132 = Not Equal?(x=w355, y=T3."Closed" ("Front Panel Window:State")) -> (x != y?=w354:bool)
            n133 = case shown="True" w354 {
              tunnel: [w362 w365] -> w361
              tunnel: w359 -> [w362 w364]
              tunnel: w357 -> [_ w363]
              frame False {
              }
              frame True {
                n134 = invoke class="VI" method="FP.Close"(reference=w363, error in=w364) -> (error out=w365:errorcluster)  [unwired: 1 in, 2 out]
              }
            }
          }
          frame "Hidden", "Hide" {
            w366 = T3."Hidden" ("State")
            n135 = property class="VI"(reference=w372, error in=w371) -> (reference out=w369:refnum<vi>, error out=w370:errorcluster, "FP.State"=w368:T3)
            n136 = Not Equal?(x=w368, y=w366) -> (x != y?=w367:bool)
            n137 = case shown="True" w367 {
              tunnel: [w377 w378] -> w373
              tunnel: w370 -> [w376 w378]
              tunnel: w369 -> [w375 _]
              tunnel: w366 -> [w374 _]
              frame True {
                n138 = invoke class="VI" method="FP.Open"(reference=w375, error in=w376, "State"=w374) -> (error out=w377:errorcluster)  [unwired: 2 in, 4 out]
              }
              frame False {
              }
            }
          }
          frame "Minimize", "Minimized" {
            w379 = T3."Minimized" ("State")
            n139 = property class="VI"(reference=w385, error in=w384) -> (reference out=w382:refnum<vi>, error out=w383:errorcluster, "FP.State"=w381:T3)
            n140 = Not Equal?(x=w381, y=w379) -> (x != y?=w380:bool)
            n141 = case shown="True" w380 {
              tunnel: [w390 w391] -> w386
              tunnel: w383 -> [w389 w391]
              tunnel: w382 -> [w388 _]
              tunnel: w379 -> [w387 _]
              frame True {
                n142 = invoke class="VI" method="FP.Open"(reference=w388, error in=w389, "State"=w387) -> (error out=w390:errorcluster)  [unwired: 2 in, 4 out]
              }
              frame False {
              }
            }
          }
          frame "Maximize", "Maximized" {
            w392 = T3."Maximized" ("State")
            n143 = property class="VI"(reference=w398, error in=w397) -> (reference out=w395:refnum<vi>, error out=w396:errorcluster, "FP.State"=w394:T3)
            n144 = Not Equal?(x=w394, y=w392) -> (x != y?=w393:bool)
            n145 = case shown="True" w393 {
              tunnel: [w403 w404] -> w399
              tunnel: w396 -> [w402 w404]
              tunnel: w395 -> [w401 _]
              tunnel: w392 -> [w400 _]
              frame True {
                n146 = invoke class="VI" method="FP.Open"(reference=w401, error in=w402, "State"=w400) -> (error out=w403:errorcluster)  [unwired: 2 in, 4 out]
              }
              frame False {
              }
            }
          }
        }
        n147 = call <vilib>:"Add State(s) to Queue__JKI_lib_State_Machine.vi"("State(s) in (\"\")"=w339) -> ("States Out"=w338:string)  [unwired: 14 in]
      }
      frame "UI: Change Waveform Graph Legend Num" {
        n148 = Unbundle By Name(w411) -> ("UI Refs.Data Ref"=w410:refnum<vi>)
        n149 = call "Convert API String Arguments to Data.vim"("Reference Type"=u32 0 ("Legend:Number of Rows"), "API String"=w408) -> ("error out"=w406:errorcluster, "Data"=w409:u32)  [unwired: 6 in]
        n150 = property class="WFChart (strict)"(reference=w410, error in=w406, "LegNumRows"=w409) -> (error out=w405:errorcluster)  [unwired: 1 out]
      }
      frame "UI: Update Waveform Graph" {
        n151 = call "CSM - Convert Argument to MassData.vim"("Type"=waveform(dbl)[] [] ("Data"), "MassData Argument"=w426) -> ("error out"=w424:errorcluster, "Data"=w420:waveform(dbl)[])  [unwired: 6 in]
        "WaveformGraph" <- w420
        n152 = Array Size(array=w420) -> (size(s)=w417:i32)
        n153 = feedback-in #1(w417) -> ()
        n154 = feedback #1(0) -> (w418:i32)
        n155 = Not Equal?(x=w417, y=w418) -> (x != y?=w414:bool)
        n156 = Format Into String(w417) -> (resulting string=w419:string)  [unwired: 3 in, 1 out]
        n157 = call <vilib>:"Build State String with Arguments__JKI_lib_State_Machine.vi"("Arguments (\"\")"=w419, "State"="UI: Change Waveform Graph Legend Num") -> ("State with Arguments"=w415:string)  [unwired: 4 in]
        n158 = call-poly <userlib>:"Add State(s) to Queue By BOOL++.vi"("TRUE (\"\")"=w415, "Condition"=w414, "State Queue (\"\")"=w422) -> ("Remaining States"=w423:string)  [unwired: 8 in]
      }
      frame "UI: Update AnalysisWnd 1" {
        n159 = call "CSM - Convert Argument to MassData.vim"("Type"=cluster{"f0":dbl, "df":dbl, "magnitude":dbl[]}[] [] ("FFT - (RMS)"), "MassData Argument"=w432) -> ("error out"=w431:errorcluster, "Data"=→"AnalysisWnd 1":cluster{"f0":dbl, "df":dbl, "magnitude":dbl[]}[])  [unwired: 6 in]
      }
      frame "UI: Update AnalysisWnd 2" {
        n160 = call "CSM - Convert Argument to MassData.vim"("Type"=cluster{"f0":dbl, "df":dbl, "magnitude":dbl[]}[] [] ("FFT - (RMS)"), "MassData Argument"=w439) -> ("error out"=w438:errorcluster, "Data"=→"AnalysisWnd 2":cluster{"f0":dbl, "df":dbl, "magnitude":dbl[]}[])  [unwired: 6 in]
      }
      frame "---------- Macro ----------" {
        n161 = call <vilib>:"Add State(s) to Queue__JKI_lib_State_Machine.vi"("State(s) in (\"\")"=w447) -> ("States Out"=w446:string)  [unwired: 14 in]
      }
      frame "Macro: Initialize" {
        w448 = "Data: Initialize\nInitialize Core Data\nEvents: Register\nUI: Initialize\nUI: Front Panel State >> Open\nUI: Change Waveform Graph Legend Num >> 1\nDO: Update Status >> Ready...\n\n//Permanent registrations\nAcquired Waveform@Acquisition >> API: Log@Logging -><register>\nAcquired Waveform@Acquisition >> UI: Update Waveform Graph -><register>\n\n//Dynamic registrations\nMacro: Register Analysis Relationships\n\n//Launch Acquisition Module\nMacro: Launch Acquisition Module"  # Data: Initialize Initialize Core Data Events: Register UI: Initialize UI: Front Panel State >> Open UI: Change Waveform Graph Legend Num >> 1 DO: Update Status >> Ready...  //Permanent registrations Acquired Waveform@Acquisition >> API: Log@Logging -><register> Acquired Waveform@Acquisition >> UI: Update Waveform Graph -><register>  //Dynamic registrations Macro: Register Analysis Relationships  //Launch Acquisition Module Macro: Launch Acquisition Module
        # "Initialization Macro\n(This is called once, when the VI starts)"
        n162 = call <userlib>:"CSM - Populate Configuration Variables.vi"("String with INI-Variable"=w448) -> ("String"=w449:string)  [unwired: 7 in, 1 out]
        n163 = call <vilib>:"Add State(s) to Queue__JKI_lib_State_Machine.vi"("State(s) in Front (\"\")"=w449, "State(s) in (\"\")"=w454) -> ("States Out"=w453:string)  [unwired: 13 in]
      }
      frame "Macro: Launch Acquisition Module" {
        n164 = local read "Data Source"() -> (w457:enum16{"Simulated Waveform", "Sound Card"})
        n165 = case shown="\"Simulated Waveform\", Default" w457 {
          tunnel: ["Do: Launch Simulated Acquisition Module" ("State(s) in (\"\")") "Do: Launch Sound Card Acquisition Module" ("State(s) in (\"\")")] -> w456
          frame "Simulated Waveform", Default {
          }
          frame "Sound Card" {
          }
        }
        n166 = call <vilib>:"Add State(s) to Queue__JKI_lib_State_Machine.vi"("State(s) in (\"\")"="Do: Exit Acquisition Module If Exist" ("State(s) in (\"\")"), "State(s) at Back (\"\")"=w456) -> ("States Out"=w455:string)  [unwired: 13 in]
        n167 = call <vilib>:"Add State(s) to Queue__JKI_lib_State_Machine.vi"("State(s) in Front (\"\")"=w455, "State(s) in (\"\")"=w459) -> ("States Out"=w460:string)  [unwired: 13 in]
      }
      frame "Macro: Register Analysis Relationships" {
        # "<2>"
        # "<1>"
        # "#CSM-NOTE\n<1> and <2> will be replaced."
        # "#CSM-NOTE\nState could be registered as status. It's similar to Status with response as its argument."
        n168 = Format Into String("Analysis Window 1") -> (resulting string=w467:string)  [unwired: 3 in, 1 out]
        n169 = Format Into String("Analysis Window 2") -> (resulting string=w466:string)  [unwired: 3 in, 1 out]
        n170 = call-poly <userlib>:"Build Message with Arguments++.vi"("States With Replace Token"="//Dynamic registrations\n\n//For AnalysisWnd 1\nAcquired Waveform@Acquisition >> API: <1>@Algorithm -><register>\nAPI: <1>@Algorithm >> UI: Update AnalysisWnd 1 -><register>\n//For AnalysisWnd 2\nAcquired Waveform@Acquisition >> API: <2>@Algorithm -><register>\nAPI: <2>@Algorithm >> UI: Update AnalysisWnd 2 -><register>" ("State(s) in Front (\"\")"), "<1>"=w467, "<2>"=w466) -> ("States"=w470:string)  [unwired: 12 in]
        n171 = Bundle By Name(cluster=w476, "Relationships"=w470) -> (w472:T9)
        n172 = call <vilib>:"Add State(s) to Queue__JKI_lib_State_Machine.vi"("State(s) in Front (\"\")"=w470, "State(s) in (\"\")"=w473) -> ("States Out"=w474:string)  [unwired: 13 in]
      }
      frame "Macro: Unregister Analysis Relationships" {
        n173 = Unbundle By Name(w488) -> ("Relationships"=w487:string)
        n174 = Search and Replace String(replace all?=TRUE ("ignore case? (F)"), case sensitive?=TRUE ("ignore case? (F)"), input string=w487, search string="<register>" ("replace string (\"\")"), replace string="<unregister>" ("replace string (\"\")")) -> (result string=w480:string)  [unwired: 3 in, 3 out]
        n175 = Bundle By Name(cluster=w488, "Relationships"="") -> (w479:T9)
        n176 = call <vilib>:"Add State(s) to Queue__JKI_lib_State_Machine.vi"("State(s) in Front (\"\")"=w480, "State(s) in (\"\")"=w481) -> ("States Out"=w482:string)  [unwired: 13 in]
      }
      frame "Macro: Start" {
        n177 = Bundle By Name(cluster=w495, "State"=UI_State."Acquiring and Logging" ("UI State")) -> (w494:T9)
        n178 = call <vilib>:"Add State(s) to Queue__JKI_lib_State_Machine.vi"("State(s) in Front (\"\")"="//Local States\nDO: Update Status >> Acquiring and Logging...\nUI: Update When Start\n\n//Send Message to Other CSM Modules\nAPI: Start -@ Logging\nAPI: Start ->| Acquisition" ("State(s) in Front (\"\")"), "State(s) in (\"\")"=w492) -> ("States Out"=w493:string)  [unwired: 13 in]
      }
      frame "Macro: Stop" {
        n179 = Unbundle By Name(w499) -> ("State"=w501:T5)
        n180 = case shown="Default" w501 {
          selector: w501 -> [w508 _]
          tunnel: [w508 UI_State."Waiting for Stop" ("UI State")] -> w500
          frame "Waiting for Exit" {
          }
          frame Default {
          }
        }
        n181 = Bundle By Name(cluster=w499, "State"=w500) -> (w505:T9)
        n182 = call <vilib>:"Add State(s) to Queue__JKI_lib_State_Machine.vi"("State(s) in Front (\"\")"="//Local States\nDO: Update Status >> Stopping...\nUI: Update When Stop\n\n//Send Message to Other CSM Modules\nAPI: Stop -@ Acquisition\nAPI: Stop -@ Logging\n" ("State(s) in Front (\"\")"), "State(s) in (\"\")"=w503) -> ("States Out"=w504:string)  [unwired: 13 in]
      }
      frame "Macro: Exit" {
        w517 = "//UI: Front Panel State >> Close"  # //UI: Front Panel State >> Close
        w514 = "//Dynamic registrations\nMacro: Unregister Analysis Relationships\n\n//Permanent registrations\nAcquired Waveform@Acquisition >> API: Log@Logging -><unregister>\nAcquired Waveform@Acquisition >> UI: Update Waveform Graph -><unregister>\n\nData: Cleanup\nEvents: Unregister\nExit"  # //Dynamic registrations Macro: Unregister Analysis Relationships  //Permanent registrations Acquired Waveform@Acquisition >> API: Log@Logging -><unregister> Acquired Waveform@Acquisition >> UI: Update Waveform Graph -><unregister>  Data: Cleanup Events: Unregister Exit
        # "Exit Macro\n(This is called once, when the VI exits)"
        n183 = Unbundle By Name(w519) -> ("Core.Close Panel on Exit?"=w518:bool)
        n184 = disable-structure shown="Enabled" {
          disable-tunnel: [w522 w534 w540] -> w511
          disable-tunnel: w510 -> [_ w533 _]
          frame Disabled {
            w529 = "Macro: Exit -@ Acquisition\nMacro: Exit -@ Logging"  # Macro: Exit -@ Acquisition Macro: Exit -@ Logging
            n185 = call <userlib>:"CSM - Module Status.vi"("CSM Name"="Algorithm") -> ("#Nodes"=w525:i32, "CSM Name (Dup)"=w527:string)  [unwired: 6 in, 3 out]
            n186 = for {
              N: w525 -> [_]
              tunnel: w527 -> [w532]
              tunnel: "Macro: Exit" -> [w531]
              tunnel: [w530] -> w523 mode=indexing
              n187 = call-poly <userlib>:"Build Message with Arguments++.vi"("State With Arguments"=w531, "Target Module (\"\")"=w532) -> ("CSM Message String"=w530:string)  [unwired: 13 in]
            }
            n188 = Build Array (concatenate)(w529, w523) -> (w524:string[])
            n189 = call <userlib>:"CSM - Compact Multiple States.vi"("Multiple States"=w524) -> ("States"=w522:string)  [unwired: 9 in]
          }
          frame Enabled {
            # "#NOTE\nHelper VI is equivalent to other case"
            n190 = call <userlib>:"CSM - List Modules.vi"() -> ("Module Names"=w536:string[])  [unwired: 10 in, 1 out]
            n191 = Search 1D Array(1D array=w536, element=w533) -> (index of element=w537:i32)  [unwired: 1 in]
            n192 = Delete From Array(array=w536, index=w537) -> (array with subset deleted=w535:string[])  [unwired: 1 in, 1 out]
            n193 = call <userlib>:"CSM - Build Exit Messages of CSMs.vi"("State With Arguments (\"Macro: Exit“)"="Macro: Exit" ("State with Arguments(\"Macro: Exit“)"), "CSMs"=w535) -> ("States"=w534:string)  [unwired: 13 in]
          }
          frame Disabled {
            # "#NOTE\nHelper VI is equivalent to other case"
            n194 = call <userlib>:"CSM - Build Exit Messages of CSMs.vi"("State With Arguments (\"Macro: Exit“)"="Macro: Exit" ("State with Arguments(\"Macro: Exit“)"), "CSMs"=string[] ["Acquisition", "Logging", "Algorithm"]) -> ("States"=w540:string)  [unwired: 13 in]
          }
        }
        n195 = Select(t=w517, s=w518, f="") -> (s? t:f=w515:string)
        n196 = call <vilib>:"Add State(s) to Queue__JKI_lib_State_Machine.vi"("State(s) in Front (\"\")"=w511, "State(s) in (\"\")"=w515, "State(s) at Back (\"\")"=w514) -> ("States Out"=w513:string)  [unwired: 12 in]
        n197 = call <vilib>:"Add State(s) to Queue__JKI_lib_State_Machine.vi"("State(s) in Front (\"\")"=w513, "State(s) in (\"\")"=w521) -> ("States Out"=w520:string)  [unwired: 13 in]
      }
      frame "---------- DoSth ----------" {
        n198 = call <vilib>:"Add State(s) to Queue__JKI_lib_State_Machine.vi"("State(s) in (\"\")"=w546) -> ("States Out"=w545:string)  [unwired: 14 in]
      }
      frame "Do: Update Status" {
        n199 = call <vilib>:"Add State(s) to Queue__JKI_lib_State_Machine.vi"("State(s) in (\"\")"=w552) -> ("States Out"=w551:string)  [unwired: 14 in]
        "Status" <- w547
      }
      frame "Do: Launch Settings Dialog" {
        # "Your code here.\n(You can make a copy of, or modify, this frame)"
        n200 = call <userlib>:"CSM - Check If Module Exists.vi"("CSM Name"="Acquisition" ("Name(\"\" to use uuid)")) -> ("error out"=w559:errorcluster, "Exist?"=w555:bool, "CSM Name (Dup)"=w557:string)  [unwired: 8 in]
        n201 = case shown="True" w555 {
          tunnel: w559 -> [w567 w579]
          tunnel: w557 -> [w563 w578]
          tunnel: w556 -> [_ w577]
          tunnel: [w566 w576] -> w554
          frame False {
            n202 = Format Into String(format string="Cannot Find the CSM which named %s !!!", w563) -> (resulting string=w562:string)  [unwired: 2 in, 1 out]
            n203 = Bundle By Name(cluster=w567, "status"=TRUE, "source"=w562) -> (w566:errorcluster)
          }
          frame True {
            w571 = T3."Standard" ("State")
            n204 = call <userlib>:"CSM - Module VI Reference.vi"("Current Module (\"\" to Generate an ID)"=w577, "error in (no error)"=w579, "Force? (F)"=TRUE ("force?(F)"), "CSM Name"=w578) -> ("error out"=w569:errorcluster, "CSM Module VIRef"=w570:refnum<vi>)  [unwired: 6 in]
            n205 = property class="VI"(reference=w570, error in=w569) -> (reference out=w574:refnum<vi>, error out=w575:errorcluster, "FP.State"=w573:T3)
            n206 = Not Equal?(x=w573, y=w571) -> (x != y?=w572:bool)
            n207 = case shown="True" w572 {
              tunnel: [w586 w588] -> w576
              tunnel: w575 -> [w581 w588]
              tunnel: w574 -> [w580 _]
              tunnel: w571 -> [w585 _]
              frame True {
                n208 = property class="VI"(reference=w580, error in=w581, "FP.Behavior"=T6."Modal" ("Front Panel Window:Behavior")) -> (reference out=w583:refnum<vi>, error out=w584:errorcluster)
                n209 = invoke class="VI" method="FP.Open"(reference=w583, error in=w584, "Activate"=TRUE, "State"=w585) -> (error out=w586:errorcluster)  [unwired: 1 in, 4 out]
              }
              frame False {
              }
            }
          }
        }
      }
      frame "Do: Confirm Quit" {
        n210 = Unbundle By Name(w593) -> ("State"=w596:T5)
        n211 = case shown="\"Acquiring and Logging\"" w596 {
          tunnel: [UI_State."Idle" ("UI State") w605] -> w595
          tunnel: w593 -> [w600 w604]
          tunnel: [w600 w603] -> w594
          tunnel: [TRUE w602] -> w589
          frame Default {
          }
          frame "Acquiring and Logging" {
            n212 = Two Button Dialog(message="Are you sure you want to quit while the acquisition is running?" ("Confirm Quit Message"), 1:"No" ("No"), 2:"Yes" ("Yes")) -> (T button?=w606:bool)
            n213 = case shown="False" w606 {
              tunnel: [UI_State."Acquiring and Logging" ("UI State") UI_State."Waiting for Exit" ("UI State")] -> w605
              tunnel: w604 -> [w610 w613]
              tunnel: [w610 w613] -> w603
              tunnel: [_ TRUE] -> w602
              frame False {
                # "User did not want to quit."
              }
              frame True {
              }
            }
          }
        }
        n214 = Bundle By Name(cluster=w594, "State"=w595) -> (w592:T9)
        n215 = call-poly <userlib>:"Add State(s) to Queue By BOOL++.vi"("TRUE (\"\")"="Macro: Exit", "Condition"=w589, "State Queue (\"\")"=w598) -> ("Remaining States"=w591:string)  [unwired: 8 in]
      }
      frame "Do: Exit Acquisition Module If Exist" {
        n216 = call <userlib>:"CSM - Check If Module Exists.vi"("CSM Name"="Acquisition") -> ("error out"=w619:errorcluster, "Exist?"=w616:bool, "CSM Name (Dup)"=w617:string)  [unwired: 8 in]
        n217 = case shown="True" w616 {
          tunnel: w619 -> [w624 w629]
          tunnel: w618 -> [_ w628]
          tunnel: w617 -> [_ w626]
          tunnel: [w624 w625] -> w615
          frame False {
          }
          frame True {
            n218 = call <userlib>:"CSM - Send Message and Wait for Reply.vi"("Current Module (\"\" to Generate an ID)"=w628, "Error In (No Error)"=w629, "Target Module"=w626, "State"="Macro: Exit") -> ("error out"=w625:errorcluster)  [unwired: 5 in, 2 out]
          }
        }
      }
      frame "Do: Launch Simulated Acquisition Module" {
        w630 = "Acquisition"  # Name("" to use uuid)
        n219 = vi-ref "Acquisition.lvlib:Acquisition.vi"() -> (w634:refnum<vi>)
        n220 = property class="VI Interface Type 5"(reference=w634) -> (reference out=w638:refnum<vi>, error out=w636:errorcluster, "Path"=w635:path)  [unwired: 1 in]
        n221 = Open VI Reference(type specifier VI Refnum (for type only)=w638, vi path=w635, options=128, error in (no error)=w636) -> (vi reference=w637:refnum<vi>, error out=w633:errorcluster)  [unwired: 2 in]
        n222 = call-by-ref "Start Asynchronous Call"(reference=w637, error in=w633, "Name(\"\" to use uuid)"=w630) -> (reference out=w640:refnum<vi>, error out=w639:errorcluster)  [unwired: 11 in]
        n223 = Close Reference(reference=w640, error in (no error)=w639) -> (error out=w632:errorcluster)
        n224 = call <userlib>:"CSM - Wait for Module to Be Alive.vi"("CSM Name"=w630, "error in (no error)"=w632) -> ("error out"=w631:errorcluster)  [unwired: 11 in, 2 out]
      }
      frame "Do: Launch Sound Card Acquisition Module" {
        w645 = "Acquisition"  # Name("" to use uuid)
        n225 = vi-ref "SoundInput-DAQ.lvlib:SoundInput-DAQ.vi"() -> (w649:refnum<vi>)
        n226 = property class="VI Interface Type 5"(reference=w649) -> (reference out=w653:refnum<vi>, error out=w651:errorcluster, "Path"=w650:path)  [unwired: 1 in]
        n227 = Open VI Reference(type specifier VI Refnum (for type only)=w653, vi path=w650, options=128, error in (no error)=w651) -> (vi reference=w652:refnum<vi>, error out=w648:errorcluster)  [unwired: 2 in]
        n228 = call-by-ref "Start Asynchronous Call"(reference=w652, error in=w648, "Name(\"\" to use uuid)"=w645) -> (reference out=w655:refnum<vi>, error out=w654:errorcluster)  [unwired: 11 in]
        n229 = Close Reference(reference=w655, error in (no error)=w654) -> (error out=w647:errorcluster)
        n230 = call <userlib>:"CSM - Wait for Module to Be Alive.vi"("CSM Name"=w645, "error in (no error)"=w647) -> ("error out"=w646:errorcluster)  [unwired: 11 in, 2 out]
      }
    }
  }
  n231 = call <userlib>:"CSM - Sync Configuration Variables to File.vi"("All Temp Variable to Default Ini(F)"=TRUE, "error in (no error)"=w2) -> ("error out"=w1:errorcluster)  [unwired: 7 in]
  n232 = disable-structure shown="RUN_TIME_ENGINE==True" {
    disable-tunnel: w1 -> [_ _]
    frame condition #0 (active) {
    }
    frame condition #1 {
      n233 = Quit LabVIEW(quit? (T)=TRUE) -> ()
    }
  }
